vi "OS Prompt.vi"(8 "error":errorcluster, 10 "SDO object in":refnum<k20>, 11 "String":string) -> (0 "error out":errorcluster)   [LabVIEW 2014]
uses:
  <vilib>/CANopenLib/CANOPEN.llb/CANopen SDO Write [U8].vi
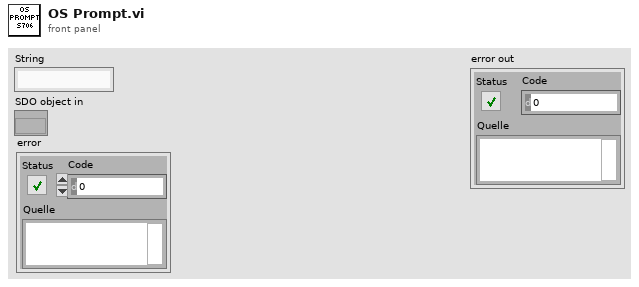
[diagram p1: front panel]
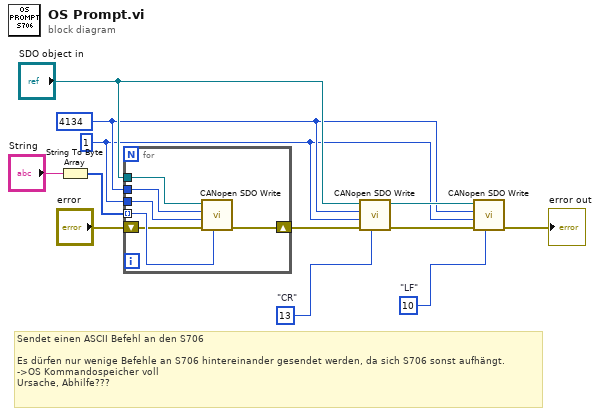
[diagram p0: block diagram]
diagram:
  w1 = u8 10  # "LF"
  w2 = u8 13  # "CR"
  w3 = u8 1 ("object sub-index (0)")
  w4 = u16 4134 ("object index")
  # "Sendet einen ASCII Befehl an den S706\n\nEs dürfen nur wenige Befehle an S706 hintereinander gesendet werden, da sich S706 sonst aufhängt.\n->OS Kommandospeicher voll\nUrsache, Abhilfe???"
  n1 = String To Byte Array(string="String") -> (unsigned byte array=w12:u8[])
  n2 = for {
    tunnel: w12 -> [w18] mode=indexing
    tunnel: "SDO object in" -> [w13]
    shift-right: [w16] -> w5
    shift-left: "error" -> [w17]
    tunnel: w4 -> [w15]
    tunnel: w3 -> [w14]
    n3 = call-poly <vilib>:"CANopen SDO Write.vi"("U8 data"=w18, "error in (no error)"=w17, "object sub-index (0)"=w14, "object index"=w15, "SDO object in"=w13) -> ("error out"=w16:errorcluster)  [unwired: 4 in, 2 out]
  }
  n4 = call-poly <vilib>:"CANopen SDO Write.vi"("U8 data"=w2, "error in (no error)"=w5, "object sub-index (0)"=w3, "object index"=w4, "SDO object in"="SDO object in") -> ("error out"=w6:errorcluster, "SDO object out"=w7:refnum<k20>)  [unwired: 4 in, 1 out]
  n5 = call-poly <vilib>:"CANopen SDO Write.vi"("U8 data"=w1, "error in (no error)"=w6, "object sub-index (0)"=w3, "object index"=w4, "SDO object in"=w7) -> ("error out"=→"error out":errorcluster)  [unwired: 4 in, 2 out]
